vi "Load Config.vi"(8 "error in (no error)":errorcluster, 11 "Role Manager in":refnum<class "Role Manager.lvclass">) -> (0 "error out":errorcluster, 3 "Role Manager out":refnum<class "Role Manager.lvclass">)   [LabVIEW 2020, in "Volatus.lvlib" / "Role Manager.lvclass"]
uses:
  Role Manager.lvclass
  C:/dev/lv20CE/relink/lv-volatus/Volatus/Module/Module.lvclass
  VolatusConfig/Meta Type.ctl
  Role.ctl
  Module/Module.lvclass/Module.ctl
  VolatusConfig/VolatusConfigElement/VolatusConfigElement.lvclass/VolatusConfigElement.ctl
  Role Manager.lvclass/Role Manager.ctl
  Module/Config.vi
  VolatusConfig/VolatusConfigElement/Element.vi
  VolatusConfig/Task/Task Config.lvclass
  C:/dev/lv20CE/relink/lv-volatus/VolatusConfig/VolatusConfigElement/VolatusConfigElement.lvclass
  lv-cdm/CDM-Config/Config Lookup/Match Meta.vi
  lv-cdm/CDM-Config/Config Element/Owner.vi
  lv-cdm/CDM-Config/Config Filter/Config Lookup.lvclass
  Module/Module.lvclass
  VolatusConfig/VolatusConfigElement/VolatusConfigElement.lvclass
  VolatusConfig/VolatusConfig.lvlib
  lv-cdm/CDM-Config/Config Element/Config Element.lvclass
  Volatus.lvlib
  C:/dev/lv20CE/relink/lv-volatus/Volatus/Role Manager/Role Manager.lvclass
  C:/dev/lv20CE/relink/lv-volatus/VolatusConfig/Task/Task Config.lvclass
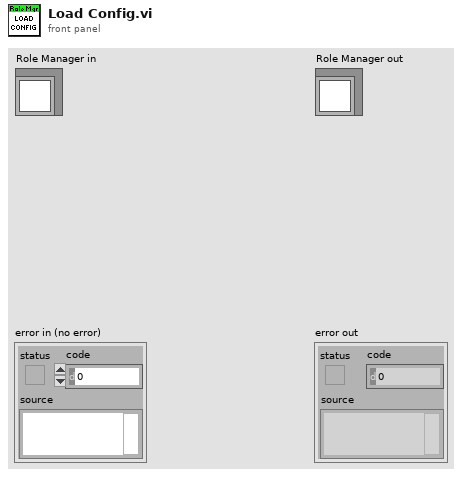
[diagram p1: front panel]
types:
  T1 = typedef "Volatus.lvlib/Role.ctl" = cluster{"Name":string, "Inherits":string[], "Hidden":bool}
  T2 = typedef "VolatusConfig.lvlib/Meta Type.ctl" = enum16{"UNKNOWN", "VL_System", "VL_Cluster", "VL_Node", "VL_Task", "VL_Group", "VL_Channel", "VL_Task_List", "VL_Scaling", "VL_Sensor", "VL_Sensor_List", "VL_Scale"}
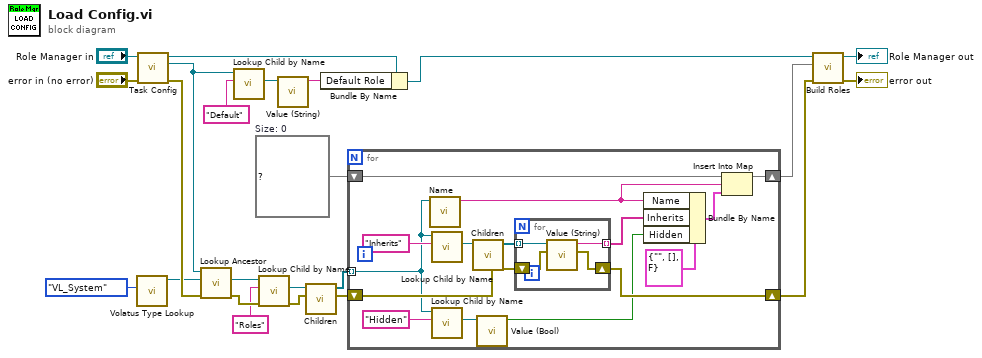
[diagram p0: block diagram]
diagram:
  w8 = map{string, T1} {}  # Size: 0
  n1 = call "Volatus Type Lookup.vi"("Meta Type"=Meta_Type."VL_System") -> ("Config Lookup out"=w18:refnum<class "Config Lookup.lvclass">)  [unwired: 9 in, 1 out]
  n2 = call "Task Config.vi"("error in (no error)"="error in (no error)", "Module in"="Role Manager in") -> ("error out"=w22:errorcluster, "Task Config"=w2:refnum<class "Task Config.lvclass">, "Module out"=w12:refnum<class "Role Manager.lvclass">)  [unwired: 7 in]
  n3 = call "Lookup Ancestor.vi"("error in (no error)"=w22, "Lookup"=w18, "VolatusConfigElement in"=w2) -> ("error out"=w23:errorcluster, "Ancestor"=w1:refnum<class "Config Element.lvclass">)  [unwired: 6 in, 1 out]
  n4 = call "Lookup Child by Name.vi"("Child Name"="Default" ("Name"), "VolatusConfigElement in"=w2) -> ("Child"=w5:refnum<class "Config Element.lvclass">)  [unwired: 6 in, 3 out]
  n5 = call "Lookup Child by Name.vi"("error in (no error)"=w23, "Name"="Roles", "Config Element in"=w1) -> ("error out"=w15:errorcluster, "Child"=w16:refnum<class "Config Element.lvclass">)  [unwired: 5 in, 2 out]
  n6 = call "Value (String).vi"("Config Element in"=w5) -> ("String Value"=w3:string)  [unwired: 9 in, 1 out]
  n7 = call "Children.vi"("error in (no error)"=w15, "Config Element in"=w16) -> ("error out"=w13:errorcluster, "Elements"=w14:refnum<class "Config Element.lvclass">[])  [unwired: 8 in]
  n8 = Bundle By Name(cluster=w12, "Default Role"=w3) -> (w4:refnum<class "Role Manager.lvclass">)
  n9 = for {
    tunnel: w14 -> [w31] mode=indexing
    shift-right: [w37] -> w10
    shift-left: w13 -> [w38]
    shift-right: [w24] -> w7
    shift-left: w8 -> [w27]
    n10 = call "Name.vi"("Config Element in"=w31) -> ("Name"=w25:string)  [unwired: 9 in, 1 out]
    n11 = call "Lookup Child by Name.vi"("Name"="Inherits", "Config Element in"=w31) -> ("Child"=w35:refnum<class "Config Element.lvclass">)  [unwired: 6 in, 3 out]
    n12 = call "Lookup Child by Name.vi"("Name"="Hidden", "Config Element in"=w31) -> ("Child"=w30:refnum<class "Config Element.lvclass">)  [unwired: 6 in, 3 out]
    n13 = call "Children.vi"("Config Element in"=w35) -> ("Elements"=w34:refnum<class "Config Element.lvclass">[])  [unwired: 9 in, 1 out]
    n14 = call "Value (Bool).vi"("Config Element in"=w30) -> ("Bool Value"=w29:bool)  [unwired: 9 in, 1 out]
    n15 = for {
      tunnel: w34 -> [w42] mode=indexing
      shift-right: [w40] -> w37
      shift-left: w38 -> [w41]
      tunnel: [w39] -> w28 mode=indexing
      n16 = call "Value (String).vi"("error in (no error)"=w41, "Config Element in"=w42) -> ("error out"=w40:errorcluster, "String Value"=w39:string)  [unwired: 8 in]
    }
    n17 = Bundle By Name(cluster=T1 {"Name"="", "Inherits"=[], "Hidden"=FALSE} ("Role"), "Name"=w25, "Inherits"=w28, "Hidden"=w29) -> (w26:T1)
    n18 = Insert Into Map(map in=w27, key=w25, value=w26) -> (map out=w24:map{string, T1})  [unwired: 2 out]
  }
  n19 = call "Build Roles.vi"("error in (no error)"=w10, "Roles"=w7, "Role Manager in"=w4) -> ("error out"=→"error out":errorcluster, "Role Manager out"=→"Role Manager out":refnum<class "Role Manager.lvclass">)  [unwired: 7 in]
